vi "Ref.vi"(7 "Destroy (f)":bool, 8 "error in (no error)":errorcluster) -> (0 "error out":errorcluster, 3 "CloneRegRef":refnum<data-value>)   [LabVIEW 2014]
uses:
  CloneRegistration.lvclass
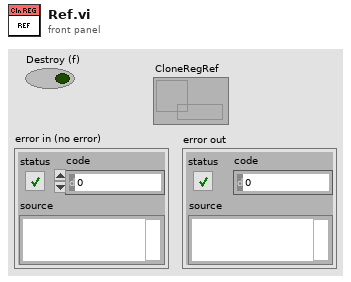
[diagram p1: front panel]
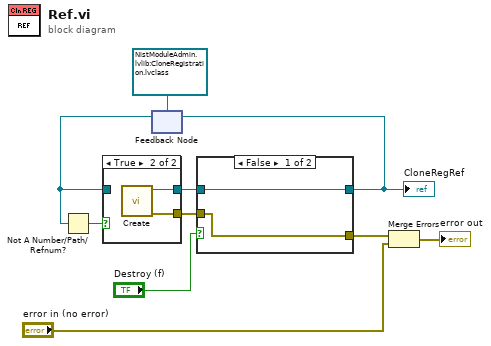
[diagram p0: block diagram]
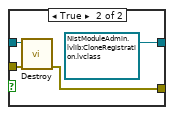
[diagram p2: hidden frame]
diagram:
  n1 = feedback #1(refnum<data-value> refnum ("CloneRegRef")) -> (w8:refnum<data-value>)
  n2 = Not A Number/Path/Refnum?(number/path/refnum=w8) -> (NaN/Path/Refnum?=w9:bool)
  n3 = case shown="True" w9 {
    tunnel: [w11 w13] -> w7
    tunnel: w8 -> [w11 _]
    tunnel: [_ w12] -> w4
    frame False {
    }
    frame True {
      n4 = call "Create.vi"() -> ("error out"=w12:errorcluster, "CloneRegRef"=w13:refnum<data-value>)  [unwired: 10 in]
    }
  }
  n5 = case shown="False" "Destroy (f)" {
    tunnel: w7 -> [w15 w19]
    tunnel: [w15 refnum<data-value> refnum ("CloneRegRef")] -> w5
    tunnel: w4 -> [w14 w17]
    tunnel: [w14 w16] -> w3
    frame False {
    }
    frame True {
      n6 = call "Destroy.vi"("error in (no error)"=w17, "CloneRegRef"=w19) -> ("error out"=w16:errorcluster)  [unwired: 9 in]
    }
  }
  "CloneRegRef" <- w5
  n7 = feedback-in #1(w5) -> ()
  n8 = Merge Errors(w3, "error in (no error)") -> (→"error out":errorcluster)
